vi "Connect.vi"(8 "error in (no error)":errorcluster, 10 "URL":string, 11 "Network Actor in":refnum<class "Client Proxy LNA.lvclass">) -> (0 "error out":errorcluster, 3 "Network Actor out":refnum<class "Client Proxy LNA.lvclass">)   [LabVIEW 2017, in "Client Proxy LNA.lvlib" / "Client Proxy LNA.lvclass"]
doc: "Opens a connection to a remote Linked Network Actor reader stream, Sends a message to the remote Linked Network Actor to connect to the local reader stream."
uses:
  Client Proxy LNA.lvclass
  C:/Program Files (x86)/National Instruments/LabVIEW 2017/vi.lib/ActorFramework/Actor/Actor.lvclass
  MAL-Framework/user.lib/Common Components/Controller/Messages/Scan Hardware Message/Scan Hardware Message.lvclass
  C:/Program Files (x86)/National Instruments/LabVIEW 2017/vi.lib/ActorFramework/Message/Message.lvclass
  <vilib>/ActorFramework/Actor/Actor.lvclass/Actor.ctl
  <vilib>/ActorFramework/Message Enqueuer/Message Enqueuer.lvclass/Message Enqueuer.ctl
  <vilib>/ActorFramework/Message Enqueuer/Init from Existing Queue.vi
  <vilib>/ActorFramework/Message Enqueuer/Message Enqueuer.lvclass
  <vilib>/NI/Actors/Linked Network Actor/Linked Network Actor/Linked Network Actor.lvclass
  <vilib>/ActorFramework/Actor/Actor.lvclass
  MAL-Framework/user.lib/Common Components/Controller/Messages/Log Status/Log Status.lvclass
  <vilib>/NI/Actors/Linked Network Actor/Linked Network Actor Messages/Transmit Network Message Msg/Transmit Network Message Msg.lvclass
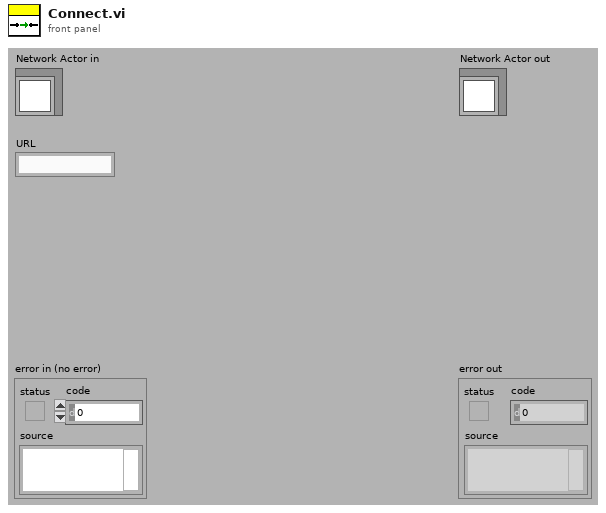
[diagram p1: front panel]
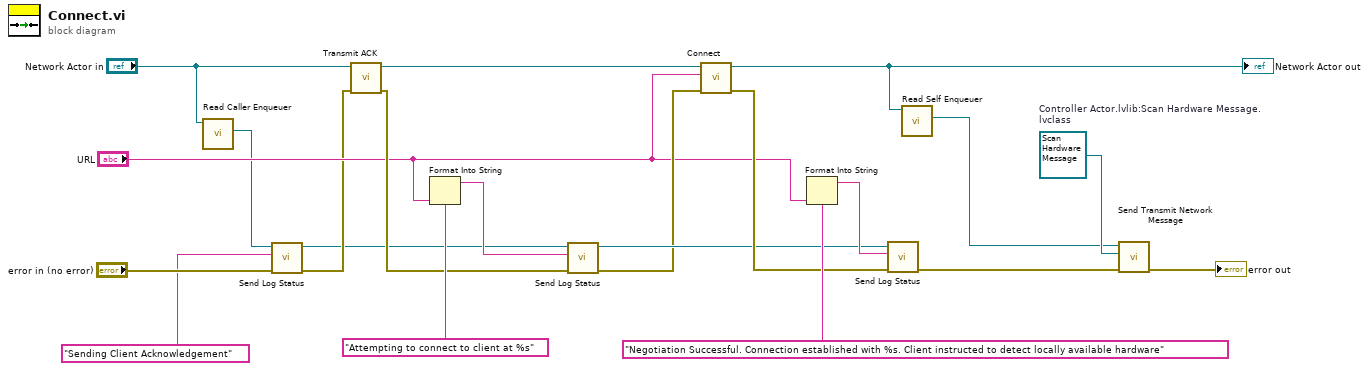
[diagram p0: block diagram]
diagram:
  w21 = refnum<class "Scan Hardware Message.lvclass"> refnum  # Controller Actor.lvlib:Scan Hardware Message.lvclass
  n1 = call <vilib>:"Read Caller Enqueuer.vi"("Actor"="Network Actor in") -> ("Caller Enqueuer"=w5:refnum<class "Message Enqueuer.lvclass">)  [unwired: 10 in]
  n2 = call "Send Log Status.vi"("error in (no error)"="error in (no error)", "String"="Sending Client Acknowledgement", "Message Enqueuer in"=w5) -> ("error out"=w3:errorcluster, "Message Enqueuer out"=w2:refnum<class "Message Enqueuer.lvclass">)  [unwired: 7 in]
  n3 = call "Transmit ACK.vi"("error in (no error)"=w3, "Client Proxy LNA in"="Network Actor in") -> ("error out"=w9:errorcluster, "Client Proxy LNA out"=w12:refnum<class "Client Proxy LNA.lvclass">)  [unwired: 8 in]
  n4 = Format Into String(format string="Attempting to connect to client at %s", "URL") -> (resulting string=w8:string)  [unwired: 2 in, 1 out]
  n5 = call "Send Log Status.vi"("error in (no error)"=w9, "String"=w8, "Message Enqueuer in"=w2) -> ("error out"=w10:errorcluster, "Message Enqueuer out"=w11:refnum<class "Message Enqueuer.lvclass">)  [unwired: 7 in]
  n6 = call-parent "Connect.vi"("error in (no error)"=w10, "URL"="URL", "Network Actor in"=w12) -> ("error out"=w15:errorcluster, "Network Actor out"=w20:refnum<class "Client Proxy LNA.lvclass">)  [unwired: 7 in]
  "Network Actor out" <- w20
  n7 = Format Into String(format string="Negotiation Successful. Connection established with %s. Client instructed to detect locally available hardware" ("string"), "URL") -> (resulting string=w16:string)  [unwired: 2 in, 1 out]
  n8 = call "Send Log Status.vi"("error in (no error)"=w15, "String"=w16, "Message Enqueuer in"=w11) -> ("error out"=w14:errorcluster)  [unwired: 7 in, 1 out]
  n9 = call <vilib>:"Read Self Enqueuer.vi"("Actor"=w20) -> ("Self Enqueuer"=w18:refnum<class "Message Enqueuer.lvclass">)  [unwired: 10 in]
  n10 = call <vilib>:"Send Transmit Network Message.vi"("error in (no error)"=w14, "Message"=w21, "Message Enqueuer"=w18) -> ("error out"=→"error out":errorcluster)  [unwired: 7 in, 1 out]
